vi "Get Data Type.vi"(8 "error in (no error)":errorcluster, 11 "Sub Object in":refnum<class "Sub Object.lvclass">) -> (0 "error out":errorcluster, 2 "Data Type":T1={"Data Type"=1, "Null"=TRUE} {"Data Type" items=["BOOLEAN"=1, "INTEGER8"=2, "INTEGER16"=3, "INTEGER32"=4, "UNSIGNED8"=5, "UNSIGNED16"=6, "UNSIGNED32"=7, "REAL32"=8, "VISIBLE_STRING"=9, "OCTET_STRING"=10, "UNICODE_STRING"=11, "TIME_OF_DAY"=12, "TIME_DIFFERENCE"=13, "RESERVED1"=14, "DOMAIN"=15, "INTEGER24"=16, "REAL64"=17, "INTEGER40"=18, "INTEGER48"=19, "INTEGER56"=20, "INTEGER64"=21, "UNSIGNED24"=22, "RESERVED2"=23, "UNSIGNED40"=24, "UNSIGNED48"=25, "UNSIGNED56"=26, "UNSIGNED64"=27, "RESERVED3"=28, "RESERVED4"=29, "RESERVED5"=30, "RESERVED6"=31, "PDO_COMMUNICATION_PARAMETER"=32, "PDO_MAPPING"=33, "SDO_PARAMETER"=34, "IDENTITY"=35, "RESERVED7"=36]}, 3 "Sub Object out":refnum<class "Sub Object.lvclass">)   [LabVIEW 2019, in "Electronic Datasheet.lvlib" / "Sub Object.lvclass"]
uses:
  Sub Object.lvclass
  Sub Object.lvclass/Sub Object.ctl
  Data Type.ctl
  Electronic Datasheet.lvlib
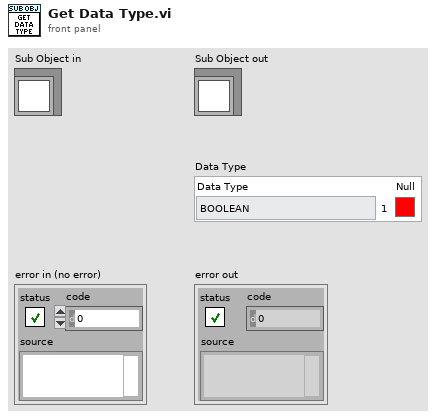
[diagram p1: front panel]
types:
  T1 = typedef "Electronic Datasheet.lvlib/Data Type.ctl" = cluster{"Data Type":u16, "Null":bool}
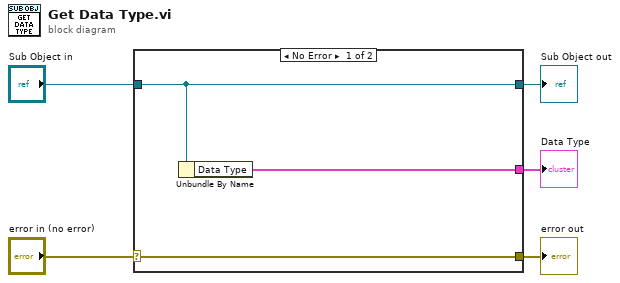
[diagram p0: block diagram]
diagram:
  n1 = case shown="No Error" "error in (no error)" {
    selector: "error in (no error)" -> [w8 w9]
    tunnel: [w8 w9] -> w4
    tunnel: [w7 w10] -> w2
    tunnel: "Sub Object in" -> [w7 w10]
    tunnel: [w6 _] -> w1
    frame No Error {
      n2 = Unbundle By Name(w7) -> ("Data Type"=w6:T1)
    }
    frame Error {
    }
  }
  "error out" <- w4
  "Sub Object out" <- w2
  "Data Type" <- w1
